vi "MRC Sim System Server Set Team.vi"(8 "error in (no error)":errorcluster, 11 "team":T1) -> (0 "error out":errorcluster)   [LabVIEW 2026, in "MrcLib.lvlib"]
doc: "MRC_Status MRC_CALLCONV MRC_SimSystemServer_SetTeam(const struct MRC_String* team);"
uses:
  MrcLib.lvlib
  <vilib>/MRC/Types/MRC String.ctl
  MrcLib.dll
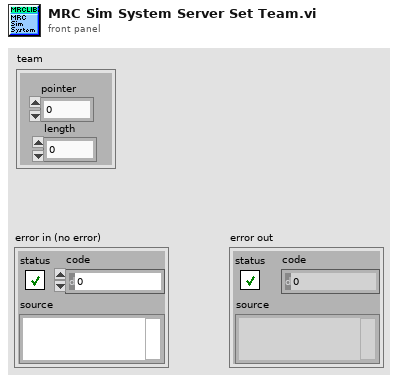
[diagram p1: front panel]
types:
  T1 = typedef "MRC String.ctl" = cluster{"pointer":u64, "length":u64}
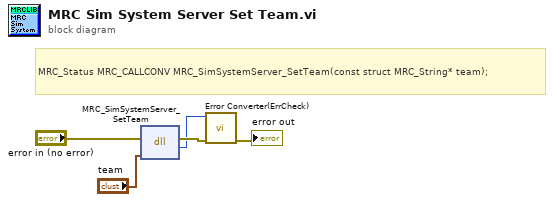
[diagram p0: block diagram]
diagram:
  # "MRC_Status MRC_CALLCONV MRC_SimSystemServer_SetTeam(const struct MRC_String* team);"
  n1 = dll-call lib="MrcLib.*" fn="MRC_SimSystemServer_SetTeam"(error in="error in (no error)", "team"="team") -> (error out=w2:errorcluster, w1:i32)  [unwired: 3 in, 1 out]
  n2 = call <vilib>:"Error Converter(ErrCheck).vi"("error in (no error)"=w2, "status"=w1) -> ("error out"=→"error out":errorcluster)  [unwired: 9 in]
